vi "Irregular Array Subset (I32).vi"(8 "Mask":bool[](array[boolean]), 10 "Array":i32[](array[numeric])) -> (0 "Indices":i32[](array[numeric]), 2 "Array Subset":i32[](array[numeric]))   [LabVIEW 2020]
doc: "Extracts the values from the input array for which the corresponding boolean inputs are TRUE."
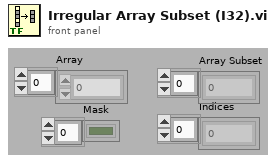
[diagram p1: front panel]
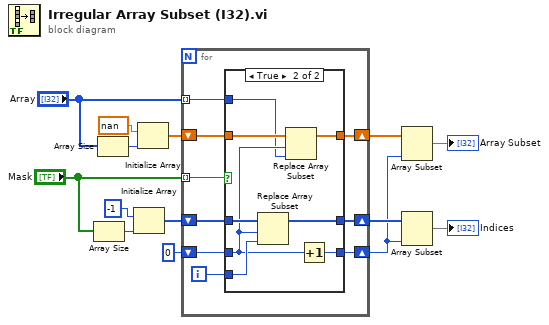
[diagram p0: block diagram]
diagram:
  n1 = Array Size(array="Mask") -> (size(s)=w14:i32)
  n2 = Array Size(array="Array") -> (size(s)=w7:i32)
  n3 = Initialize Array(-1, w14) -> (w11:i32[])
  n4 = Initialize Array(nan, w7) -> (w5:dbl[])
  n5 = for {
    tunnel: "Mask" -> [w23] mode=indexing
    shift-right: [w19] -> w9
    shift-left: w11 -> [w22]
    shift-right: [w18] -> w2
    shift-left: 0 -> [w20]
    shift-right: [w16] -> w3
    shift-left: w5 -> [w17]
    tunnel: "Array" -> [w15] mode=indexing
    i -> [w21]
    n6 = case shown="True" w23 {
      tunnel: w22 -> [w26 w34]
      tunnel: w21 -> [_ w33]
      tunnel: w20 -> [w25 w28]
      tunnel: [w25 w31] -> w18
      tunnel: [w26 w32] -> w19
      tunnel: w17 -> [w24 w30]
      tunnel: [w24 w29] -> w16
      tunnel: w15 -> [_ w27]
      frame False {
      }
      frame True {
        n7 = Replace Array Subset(array=w34, new element=w33, index=w28) -> (w32:i32[])
        n8 = Replace Array Subset(array=w30, new element=w27, index=w28) -> (w29:dbl[])
        n9 = Increment(x=w28) -> (x+1=w31:i32)
      }
    }
  }
  n10 = Array Subset(array=w3, length=w2) -> (→"Array Subset":dbl[])  [unwired: 1 in]
  n11 = Array Subset(array=w9, length=w2) -> (→"Indices":i32[])  [unwired: 1 in]
